vi "GlobalVars.vi"() -> ()   [LabVIEW 2012]
panel:
  in  "Scanning":bool
  in  "Sampling Interval (sec)":dbl
  in  "Number of Scan Planes":i32
  out "MotionAnalysis":refnum<queue>
  in  "VI Open":bool
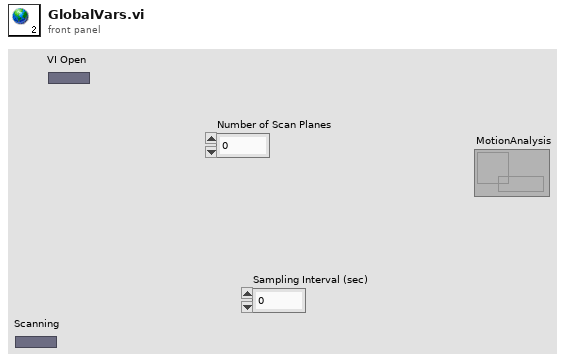
[diagram p1: front panel]
diagram:
